vi "CRYAscii Codes Decode.vi"(11 "String in, with codes":string) -> (3 "String out, decoded":string)   [LabVIEW 2013]
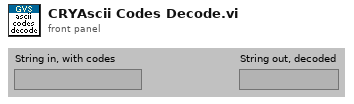
[diagram p1: front panel]
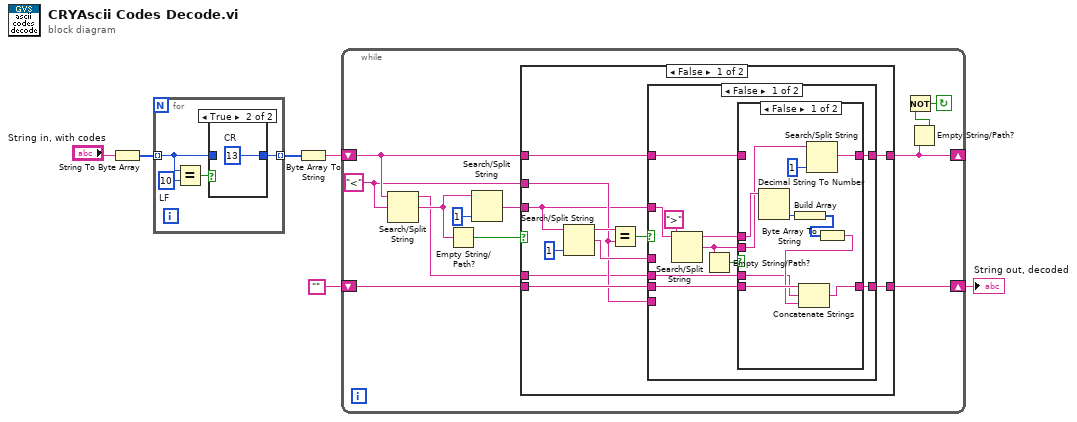
[diagram p0: block diagram]
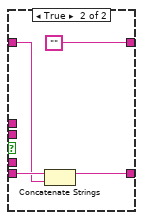
[diagram p2: hidden frame]
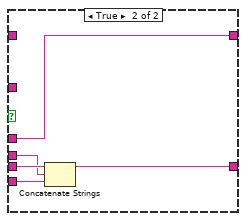
[diagram p3: hidden frame]
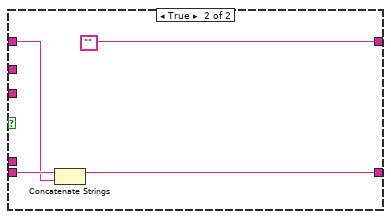
[diagram p4: hidden frame]
diagram:
  n1 = String To Byte Array(string="String in, with codes") -> (unsigned byte array=w4:u8[])
  n2 = for {
    tunnel: w4 -> [w8] mode=indexing
    tunnel: [w7] -> w3 mode=indexing
    w10 = u8 10  # LF
    n3 = Equal?(x=w8, y=w10) -> (x = y?=w9:bool)
    n4 = case shown="True" w9 {
      tunnel: [w11 w12] -> w7
      tunnel: w8 -> [w11 _]
      frame False {
      }
      frame True {
        w12 = u8 13  # CR
      }
    }
  }
  n5 = Byte Array To String(unsigned byte array=w3) -> (string=w1:string)
  n6 = while {
    shift-left: "" -> [w23]
    shift-right: [w21] -> w5
    shift-left: w1 -> [w22]
    shift-right: [w15] -> _
    stop <- w16 continue-if-true
    w13 = "<"
    n7 = Search/Split String(string=w22, search string/char (-)=w13) -> (substring before match=w17:string, match + rest of string=w19:string)  [unwired: 2 out]
    n8 = Empty String/Path?(string/path=w19) -> (empty?=w24:bool)
    n9 = Search/Split String(string=w19, offset (0)=1) -> (match + rest of string=w18:string)  [unwired: 3 out]
    n10 = case shown="False" w24 {
      tunnel: w23 -> [w30 w68]
      tunnel: w22 -> [w26 w66]
      tunnel: [w28 w67] -> w21
      tunnel: [w32 ""] -> w15
      tunnel: w18 -> [w27 _]
      tunnel: w13 -> [w29 _]
      tunnel: w17 -> [w25 _]
      frame False {
        n11 = Search/Split String(string=w27, offset (0)=1) -> (substring before match=w34:string, match + rest of string=w31:string)  [unwired: 2 out]
        n12 = Equal?(x=w34, y=w29) -> (x = y?=w33:bool)
        n13 = case shown="False" w33 {
          tunnel: [w39 w64] -> w32
          tunnel: w31 -> [_ w64]
          tunnel: w30 -> [w41 w63]
          tunnel: w29 -> [_ w61]
          tunnel: [w40 w62] -> w28
          tunnel: w27 -> [w44 _]
          tunnel: w26 -> [w42 _]
          tunnel: w25 -> [w36 w60]
          frame False {
            n14 = Search/Split String(string=w44, search string/char (-)=">") -> (substring before match=w38:string, match + rest of string=w37:string)  [unwired: 2 out]
            n15 = Empty String/Path?(string/path=w37) -> (empty?=w43:bool)
            n16 = case shown="False" w43 {
              tunnel: w42 -> [_ w57]
              tunnel: w41 -> [w52 w59]
              tunnel: [w51 w58] -> w40
              tunnel: [w48 ""] -> w39
              tunnel: w38 -> [w55 _]
              tunnel: w37 -> [w49 _]
              tunnel: w36 -> [w46 _]
              frame False {
                n17 = Decimal String To Number(string=w55) -> (number=w53:i32)  [unwired: 3 out]
                n18 = Build Array(w53) -> (w54:i32[])
                n19 = Search/Split String(string=w49, offset (0)=1) -> (match + rest of string=w48:string)  [unwired: 3 out]
                n20 = Byte Array To String(unsigned byte array=w54) -> (string=w47:string)
                n21 = Concatenate Strings(w52, w46, w47) -> (w51:string)
              }
              frame True {
                n22 = Concatenate Strings(w59, w57) -> (w58:string)
              }
            }
          }
          frame True {
            n23 = Concatenate Strings(w63, w60, w61) -> (w62:string)
          }
        }
      }
      frame True {
        n24 = Concatenate Strings(w68, w66) -> (w67:string)
      }
    }
    n25 = Empty String/Path?(string/path=w15) -> (empty?=w14:bool)
    n26 = Not(x=w14) -> (.not. x?=w16:bool)
  }
  "String out, decoded" <- w5
